vi "AddFrontPanelControls.vi"(5 "Open Front Panel":bool, 7 "Control Properties":T1[](array[typedef])=[{"label"="tag bus in ", "terminal index"=11, "indicator"=FALSE, "location"={"Horizontal"=0, "Vertical"=0}}, {"label"="tag bus out", "terminal index"=3, "indicator"=TRUE, "location"={"Horizontal"=600, "Vertical"=0}}, {"label"="cluster", "terminal index"=10, "indicator"=FALSE, "location"={"Horizontal"=200, "Vertical"=0}}, {"label"="index cluster", "terminal index"=2, "indicator"=FALSE, "location"={"Horizontal"=400, "Vertical"=0}}, {"label"="error in", "terminal index"=8, "indicator"=FALSE, "location"={"Horizontal"=0, "Vertical"=400}}, {"label"="error out", "terminal index"=0, "indicator"=TRUE, "location"={"Horizontal"=600, "Vertical"=400}}], 8 "error in":errorcluster, 11 "State":T3) -> (0 "error out":errorcluster, 2 "Terminal References":T6, 3 "State out":T3)   [LabVIEW 2013, in "data interface script.lvlib"]
uses:
  data interface script.lvlib
  Controls/TerminalReferences.ctl
  Controls/StateCluster.ctl
  Controls/initialized references.ctl
  Controls/interface VI type.ctl
  Controls/ControlsProperties.ctl
  <vilib>/Utility/miscctls.llb/LVPointTypeDef.ctl
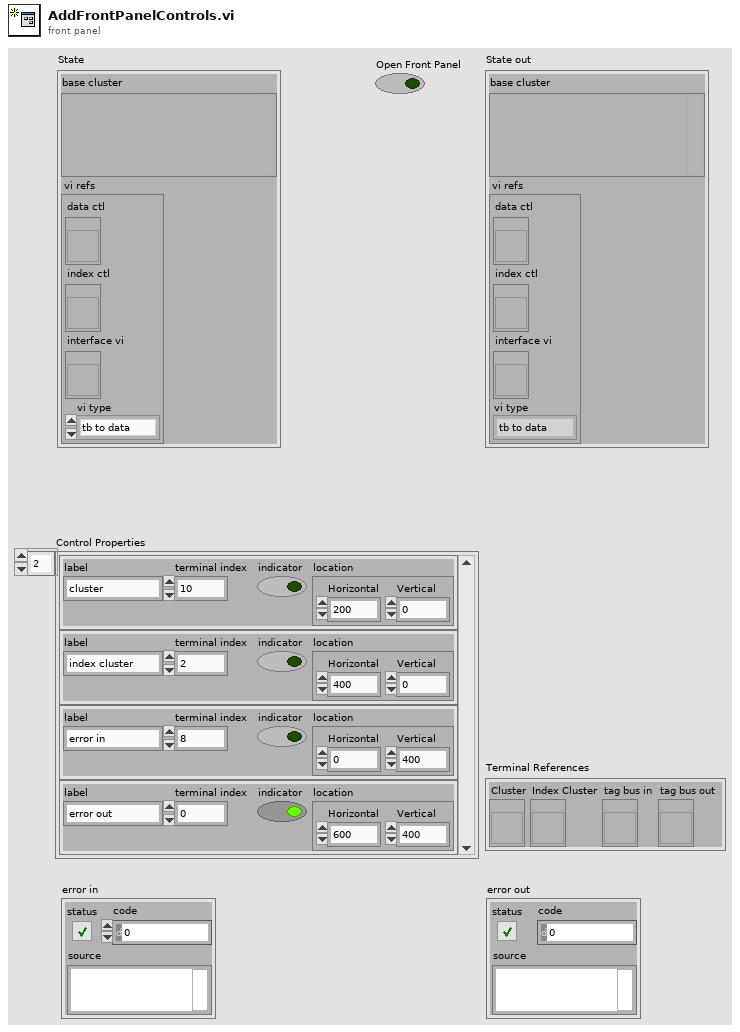
[diagram p1: front panel]
types:
  T1 = typedef "data interface script.lvlib/ControlsProperties.ctl" = cluster{"label":string, "terminal index":u32, "indicator":bool, "location":T2}
  T2 = typedef "LVPointTypeDef.ctl" = cluster{"Horizontal":i16, "Vertical":i16}
  T3 = typedef "data interface script.lvlib/StateCluster.ctl" = cluster{"base cluster":variant, "vi refs":T4}
  T4 = typedef "data interface script.lvlib/initialized references.ctl" = cluster{"data ctl":refnum<vi>, "index ctl":refnum<vi>, "interface vi":refnum<vi>, "vi type":T5}
  T5 = typedef "data interface script.lvlib/interface VI type.ctl" = enum16{"tb to data", "data to tb"}
  T6 = typedef "data interface script.lvlib/TerminalReferences.ctl" = cluster{"Cluster":refnum<vi>, "Index Cluster":refnum<vi>, "tag bus in":refnum<vi>, "tag bus out":refnum<vi>}
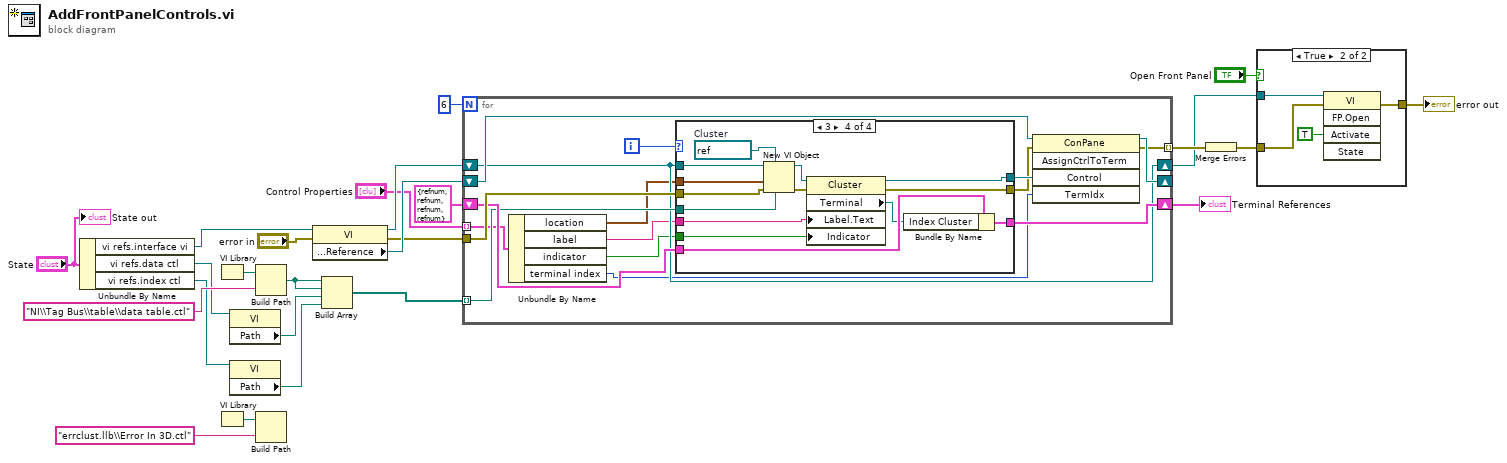
[diagram p0: block diagram]
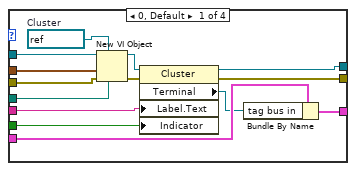
[diagram p3: hidden frame]
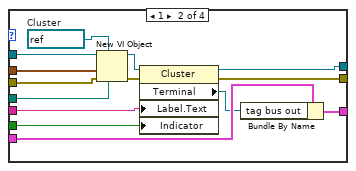
[diagram p4: hidden frame]
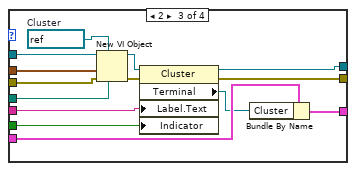
[diagram p5: hidden frame]
diagram:
  n1 = Unbundle By Name("State") -> ("vi refs.interface vi"=w3:refnum<vi>, "vi refs.data ctl"=w2:refnum<vi>, "vi refs.index ctl"=w1:refnum<vi>)
  n2 = VI Library() -> (path=w8:path)
  n3 = VI Library() -> (path=w4:path)
  n4 = property class="VI"(reference=w2) -> ("Path"=w23:path)  [unwired: 1 in, 2 out]
  n5 = property class="VI"(reference=w1) -> ("Path"=w21:path)  [unwired: 1 in, 2 out]
  n6 = Build Path(base path=w8, name or relative path="NI\\Tag Bus\\table\\data table.ctl") -> (appended path=w6:path)
  n7 = Build Path(base path=w4, name or relative path="errclust.llb\\Error In 3D.ctl") -> ()  [unwired: 1 out]
  n8 = property class="VI"(reference=w3, error in="error in") -> (reference out=w18:refnum<vi>, error out=w10:errorcluster, "Connector Pane:Reference"=w17:refnum<vi>)
  n9 = Build Array(w6, w6, w23, w21) -> (w22:path[])
  n10 = for {
    N: 6 -> [_]
    tunnel: w10 -> [w41]
    tunnel: w22 -> [w38] mode=indexing
    shift-right: [w39] -> w24
    shift-left: T6 {"Cluster"=refnum, "Index Cluster"=refnum, "tag bus in"=refnum, "tag bus out"=refnum} ("Terminal References") -> [w40]
    tunnel: [w26] -> w19 mode=indexing
    shift-right: [w34] -> _
    shift-left: w17 -> [w35]
    shift-right: [w33] -> w14
    shift-left: w18 -> [w33]
    tunnel: "Control Properties" -> [w32] mode=indexing
    i -> [w37]
    n11 = Unbundle By Name(w32) -> ("location"=w30:T2, "label"=w31:string, "indicator"=w29:bool, "terminal index"=w28:u32)
    n12 = case shown="3" w37 {
      tunnel: w41 -> [w54 w68 w82 w96]
      tunnel: w40 -> [w53 w67 w81 w95]
      tunnel: [w52 w66 w80 w94] -> w39
      tunnel: w38 -> [w50 w64 w78 w92]
      tunnel: w30 -> [w48 w62 w76 w90]
      tunnel: [w47 w61 w75 w89] -> w27
      tunnel: w33 -> [w46 w60 w74 w88]
      tunnel: w31 -> [w43 w57 w71 w85]
      tunnel: [w44 w58 w72 w86] -> w36
      tunnel: w29 -> [w42 w56 w70 w84]
      frame 0, Default {
        w55 = refnum<vi> refnum  # Cluster
        n13 = New VI Object(vi object class=w55, owner refnum=w46, position/next to=w48, 6:w50, 8:w54) -> (object refnum=w45:refnum<vi>, 0:w49:errorcluster)  [unwired: 3 in]
        n14 = property on="Property Node" class="Cluster"(reference=w45, error in=w49, "Label.Text"=w43, "Indicator"=w42) -> (reference out=w44:refnum<vi>, error out=w47:errorcluster, "Terminal"=w51:refnum<vi>)
        n15 = Bundle By Name(cluster=w53, "tag bus in"=w51) -> (w52:T6)
      }
      frame 1 {
        w69 = refnum<vi> refnum  # Cluster
        n16 = New VI Object(vi object class=w69, owner refnum=w60, position/next to=w62, 6:w64, 8:w68) -> (object refnum=w59:refnum<vi>, 0:w63:errorcluster)  [unwired: 3 in]
        n17 = property on="Property Node" class="Cluster"(reference=w59, error in=w63, "Label.Text"=w57, "Indicator"=w56) -> (reference out=w58:refnum<vi>, error out=w61:errorcluster, "Terminal"=w65:refnum<vi>)
        n18 = Bundle By Name(cluster=w67, "tag bus out"=w65) -> (w66:T6)
      }
      frame 2 {
        w83 = refnum<vi> refnum  # Cluster
        n19 = New VI Object(vi object class=w83, owner refnum=w74, position/next to=w76, 6:w78, 8:w82) -> (object refnum=w73:refnum<vi>, 0:w77:errorcluster)  [unwired: 3 in]
        n20 = property on="Property Node" class="Cluster"(reference=w73, error in=w77, "Label.Text"=w71, "Indicator"=w70) -> (reference out=w72:refnum<vi>, error out=w75:errorcluster, "Terminal"=w79:refnum<vi>)
        n21 = Bundle By Name(cluster=w81, "Cluster"=w79) -> (w80:T6)
      }
      frame 3 {
        w97 = refnum<vi> refnum  # Cluster
        n22 = New VI Object(vi object class=w97, owner refnum=w88, position/next to=w90, 6:w92, 8:w96) -> (object refnum=w87:refnum<vi>, 0:w91:errorcluster)  [unwired: 3 in]
        n23 = property on="Property Node" class="Cluster"(reference=w87, error in=w91, "Label.Text"=w85, "Indicator"=w84) -> (reference out=w86:refnum<vi>, error out=w89:errorcluster, "Terminal"=w93:refnum<vi>)
        n24 = Bundle By Name(cluster=w95, "Index Cluster"=w93) -> (w94:T6)
      }
    }
    n25 = invoke class="ConPane" method="AssignCtrlToTerm"(reference=w35, error in=w27, "Control"=w36, "TermIdx"=w28) -> (reference out=w34:refnum<vi>, error out=w26:errorcluster)  [unwired: 1 in, 3 out]
  }
  "Terminal References" <- w24
  n26 = Merge Errors(w19) -> (w13:errorcluster)
  n27 = case shown="True" "Open Front Panel" {
    tunnel: w14 -> [_ w101]
    tunnel: w13 -> [w98 w100]
    tunnel: [w98 w99] -> w12
    frame False {
    }
    frame True {
      n28 = invoke class="VI" method="FP.Open"(reference=w101, error in=w100, "Activate"=TRUE ("Activate?")) -> (error out=w99:errorcluster)  [unwired: 2 in, 4 out]
    }
  }
  "error out" <- w12
  "State out" <- "State"
